vi "if_v0_v2.vi"() -> ()   [LabVIEW 2009]
panel:
  out "Rez 2":dbl=704.4518210227099
  out "Rez1":dbl=77.5851563049165
  in  "B":dbl(knob)=77.5851563049165 scale=0.0..1000.0
  in  "A":dbl(knob)=704.4518210227099 scale=10.0..1000.0
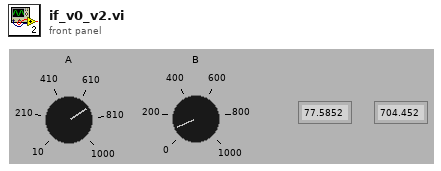
[diagram p1: front panel]
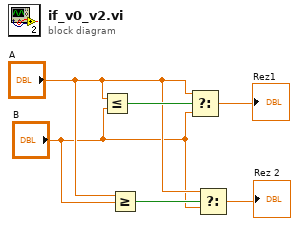
[diagram p0: block diagram]
diagram:
  n1 = Less Or Equal?(x="A", y="B") -> (x <= y?=w6:bool)
  n2 = Greater Or Equal?(x="A", y="B") -> (x >= y?=w4:bool)
  n3 = Select(t="A", s=w6, f="B") -> (s? t:f=→"Rez1":dbl)
  n4 = Select(t="A", s=w4, f="B") -> (s? t:f=→"Rez 2":dbl)
